vi "BallShooter_Execute.vi"   [LabVIEW 2020]
doc: "This routine is called every 20 milliseconds after the BEGIN routine has completed.\n\nPut code here that reads sensors, performs logic, writes to actuators."
uses:
  <vilib>/Rock Robotics/WPI/Relay/WPI_RelayValue.ctl
  <vilib>/Rock Robotics/Network Tables/NT Write Boolean.vi
types:
  T1 = typedef "WPI_SwitchDevRef.ctl" = cluster{"DevStatus":errorcluster, "DIO Channel":T2, "CntIndex":T3, "Normally Closed":bool}
  T2 = typedef "FPGA_DIOChannel.ctl" = enum8{"DIO 0", "DIO 1", "DIO 2", "DIO 3", "DIO 4", "DIO 5", "DIO 6", "DIO 7", "DIO 8", "DIO 9", "DIO MXP 0", "DIO MXP 1", "DIO MXP 2", "DIO MXP 3", "DIO MXP 4", "DIO MXP 5", "DIO MXP 6", "DIO MXP 7", "DIO MXP 8", "DIO MXP 9", "DIO MXP 10", "DIO MXP 11", "DIO MXP 12", "DIO MXP 13", "DIO MXP 14", "DIO MXP 15", "SPI Port CS1", "SPI Port CS2", "SPI Port CS3", "SPI Port MISO", "SPI Port MOSI", "Invalid"}
  T3 = typedef "FPGA_CounterCtrSystemIndex.ctl" = enum8{"Ctr 0", "Ctr 1", "Ctr 2", "Ctr 3", "Ctr 4", "Ctr 5", "Ctr 6", "Ctr 7", "Invalid"}
  T4 = typedef "WPI_RelayDevRef.ctl" = cluster{"DevStatus":errorcluster, "Relay Channel":T5, "Relay Direction":T6}
  T5 = typedef "FPGA_DIORelayChannel.ctl" = enum8{"Relay 0", "Relay 1", "Relay 2", "Relay 3", "Invalid"}
  T6 = typedef "WPI_RelayDirection.ctl" = enum16{"Both directions", "Forward only", "Reverse only"}
  T7 = typedef "WPI_DigitalOutputDevRef.ctl" = cluster{"DIO Channel":T2, "DevStatus":errorcluster}
  T8 = typedef "WPI_RelayValue.ctl" = enum16{"Off", "On", "Forward", "Reverse"}
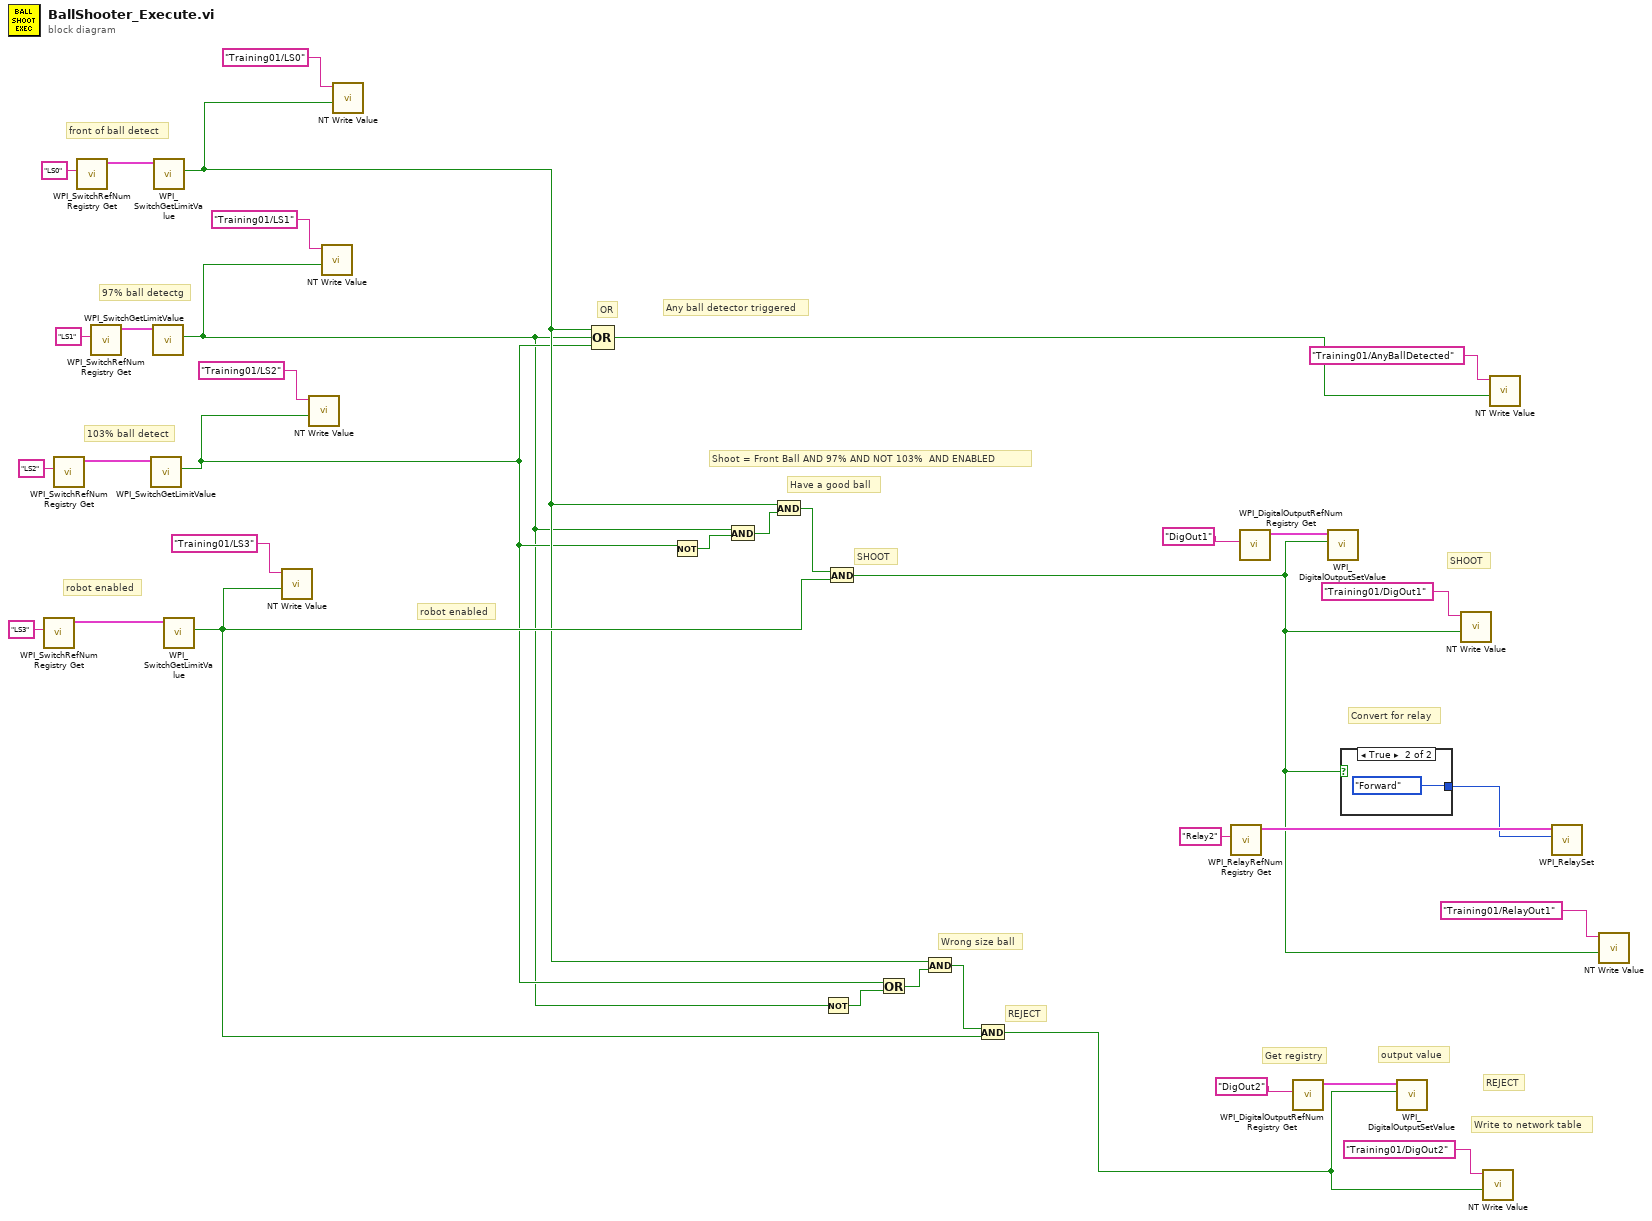
[diagram p0: block diagram]
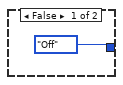
[diagram p2: hidden frame]
diagram:
  # "Write to network table"
  # "output value"
  # "Get registry"
  # "REJECT"
  # "Wrong size ball"
  # "REJECT"
  # "SHOOT"
  # "Convert for relay"
  # "SHOOT"
  # "Have a good ball"
  # "front of ball detect"
  # "97% ball detectg"
  # "103% ball detect"
  # "robot enabled"
  # "robot enabled"
  # "Shoot = Front Ball AND 97% AND NOT 103%  AND ENABLED"
  # "Any ball detector triggered"
  # "OR"
  n1 = call <vilib>:"WPI_SwitchRefNum Registry Get.vi"("refnum name"="LS3") -> ("SwitchDevRef"=w33:T1)  [unwired: 9 in, 1 out]
  n2 = call <vilib>:"WPI_SwitchRefNum Registry Get.vi"("refnum name"="LS2") -> ("SwitchDevRef"=w34:T1)  [unwired: 9 in, 1 out]
  n3 = call <vilib>:"WPI_SwitchRefNum Registry Get.vi"("refnum name"="LS0") -> ("SwitchDevRef"=w36:T1)  [unwired: 9 in, 1 out]
  n4 = call <vilib>:"WPI_SwitchRefNum Registry Get.vi"("refnum name"="LS1") -> ("SwitchDevRef"=w35:T1)  [unwired: 9 in, 1 out]
  n5 = call <vilib>:"WPI_SwitchGetLimitValue.vi"("SwitchDevRef"=w34) -> ("Switch Pressed"=w3:bool)  [unwired: 8 in, 2 out]
  n6 = call <vilib>:"WPI_SwitchGetLimitValue.vi"("SwitchDevRef"=w35) -> ("Switch Pressed"=w2:bool)  [unwired: 8 in, 2 out]
  n7 = call <vilib>:"WPI_SwitchGetLimitValue.vi"("SwitchDevRef"=w36) -> ("Switch Pressed"=w4:bool)  [unwired: 8 in, 2 out]
  n8 = call <vilib>:"WPI_SwitchGetLimitValue.vi"("SwitchDevRef"=w33) -> ("Switch Pressed"=w5:bool)  [unwired: 8 in, 2 out]
  n9 = call-poly <vilib>:"NT Write Value.vi"("value"=w5, "name"="Training01/LS3") -> ()  [unwired: 9 in, 1 out]
  n10 = call-poly <vilib>:"NT Write Value.vi"("value"=w3, "name"="Training01/LS2") -> ()  [unwired: 9 in, 1 out]
  n11 = call-poly <vilib>:"NT Write Value.vi"("value"=w2, "name"="Training01/LS1") -> ()  [unwired: 9 in, 1 out]
  n12 = call-poly <vilib>:"NT Write Value.vi"("value"=w4, "name"="Training01/LS0") -> ()  [unwired: 9 in, 1 out]
  n13 = Compound Arithmetic op=OR(w4, w2, w3) -> (w15:bool)
  n14 = Not(x=w3) -> (.not. x?=w12:bool)
  n15 = And(x=w2, y=w12) -> (x .and. y?=w13:bool)
  n16 = And(x=w4, y=w13) -> (x .and. y?=w11:bool)
  n17 = Not(x=w2) -> (.not. x?=w7:bool)
  n18 = And(x=w11, y=w5) -> (x .and. y?=w10:bool)
  n19 = Or(x=w3, y=w7) -> (x .or. y?=w8:bool)
  n20 = And(x=w4, y=w8) -> (x .and. y?=w6:bool)
  n21 = And(x=w6, y=w5) -> (x .and. y?=w1:bool)
  n22 = call <vilib>:"WPI_RelayRefNum Registry Get.vi"("refnum name"="Relay2") -> ("RelayDevRef"=w28:T4)  [unwired: 9 in, 1 out]
  n23 = call <vilib>:"WPI_DigitalOutputRefNum Registry Get.vi"("refnum name"="DigOut1") -> ("DigitalOutputDevRef"=w19:T7)  [unwired: 9 in, 1 out]
  n24 = call <vilib>:"WPI_DigitalOutputRefNum Registry Get.vi"("refnum name"="DigOut2") -> ("DigitalOutputDevRef"=w17:T7)  [unwired: 9 in, 1 out]
  n25 = call <vilib>:"WPI_DigitalOutputSetValue.vi"("Value"=w10, "DigitalOutputDevRef"=w19) -> ()  [unwired: 8 in, 2 out]
  n26 = case shown="True" w10 {
    tunnel: [WPI_RelayValue."Off" ("RelayValue") WPI_RelayValue."Forward" ("RelayValue")] -> w26
    frame False {
    }
    frame True {
    }
  }
  n27 = call <vilib>:"WPI_DigitalOutputSetValue.vi"("Value"=w1, "DigitalOutputDevRef"=w17) -> ()  [unwired: 8 in, 2 out]
  n28 = call-poly <vilib>:"NT Write Value.vi"("value"=w10, "name"="Training01/DigOut1") -> ()  [unwired: 9 in, 1 out]
  n29 = call-poly <vilib>:"NT Write Value.vi"("value"=w1, "name"="Training01/DigOut2") -> ()  [unwired: 9 in, 1 out]
  n30 = call-poly <vilib>:"NT Write Value.vi"("value"=w15, "name"="Training01/AnyBallDetected") -> ()  [unwired: 9 in, 1 out]
  n31 = call <vilib>:"WPI_RelaySet.vi"("RelayValue"=w26, "RelayDevRef"=w28) -> ()  [unwired: 8 in, 2 out]
  n32 = call-poly <vilib>:"NT Write Value.vi"("value"=w10, "name"="Training01/RelayOut1") -> ()  [unwired: 9 in, 1 out]
